vi "FTW-Ether-NewLoggerConnection.vi"(11 "error in":errorcluster) -> (4 "Event Logger Connection":refnum<class "FTW-Logger.lvclass">, 15 "error out":errorcluster)   [LabVIEW 2012, in "FTW-Actor.lvlib" / "FTW-Ether.lvclass"]
uses:
  FTW-Ether.lvclass
  EventLogger/FTW-Logger.lvclass
  FTW-Ether-Instance.vi
panel:
  # "Inputs"
  # "Outputs"
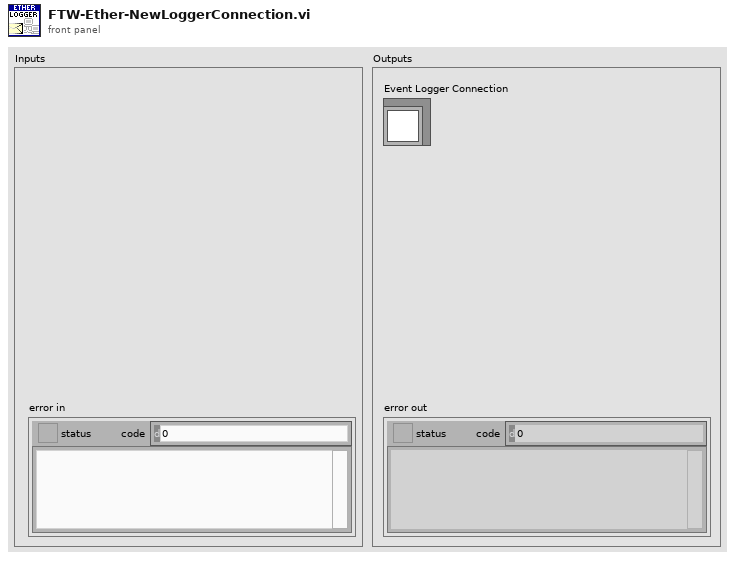
[diagram p1: front panel]
types:
  T1 = typedef "FTW-Actor.lvlib/FTW-Actor-Address.ctl" = string
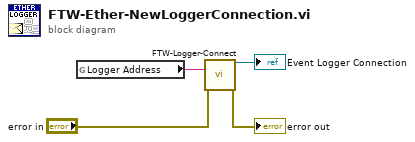
[diagram p0: block diagram]
diagram:
  n1 = global read "FTW-Ether-Instance.vi" "Logger Address"() -> (w1:T1)
  n2 = call "FTW-Logger-Connect.vi"("Logger Address"=w1, "error in"="error in") -> ("Event Logger Connection"=→"Event Logger Connection":refnum<class "FTW-Logger.lvclass">, "error out"=→"error out":errorcluster)  [unwired: 12 in]
